vi "字符补长任意.vi"(1 "in":string, 2 "长度":u8) -> (0 "out":string)   [LabVIEW 2015, in "AN97005N.lvlib"]
uses:
  AN97005N.lvlib
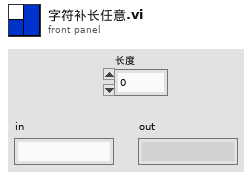
[diagram p1: front panel]
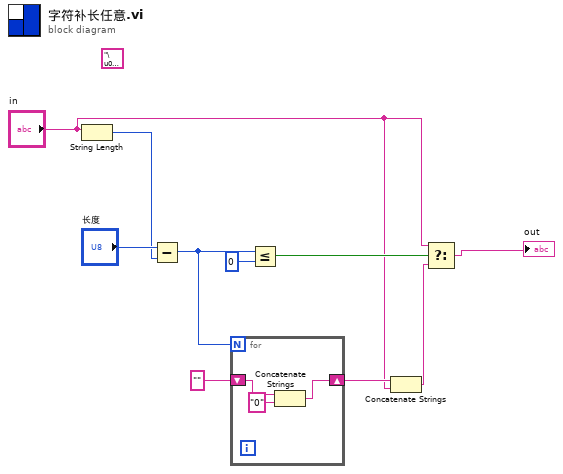
[diagram p0: block diagram]
diagram:
  (unwired) "\u0000"
  n1 = String Length(string="in") -> (length=w9:i32)
  n2 = Subtract(x="长度", y=w9) -> (x-y=w6:i32)
  n3 = for {
    N: w6 -> [_]
    shift-right: [w11] -> w4
    shift-left: "" -> [w13]
    n4 = Concatenate Strings(w13, "0" ("字符串")) -> (w11:string)
  }
  n5 = Less Or Equal?(x=w6, y=0) -> (x <= y?=w7:bool)
  n6 = Concatenate Strings(w4, "in") -> (w2:string)
  n7 = Select(t="in", s=w7, f=w2) -> (s? t:f=→"out":string)
